vi "gun_const.vi"() -> (3 "Data Out":T1={"gun"={"num_lines"=0.0, "gain_kp1"=0.0, "gain_kp2"=0.0, "gain_ki"=0.0, "gain_kd"=0.0}, "turret"={"center_ana"=0.0, "volts_per_180"=0.0, "man_scale"=0.0, "turret_idg"={"low_fault_ana"=0.0, "high_fault_ana"=0.0, "min_ana"=0.0, "max_ana"=0.0, "movement_thresh"=0.0, "movement_time"=0.0}, "turret_pid"={"kP"=0.0, "kI"=0.0, "kD"=0.0}, "turret_invert"=TRUE, "turret_low_power"=0.0}, "tracking"={"velocity_lead_gain"=0.0, "velocity_rotation_gain"=0.0}, "hood"={"hood_idg"={"low_fault_ana"=0.0, "high_fault_ana"=0.0, "min_ana"=0.0, "max_ana"=0.0, "movement_thresh"=0.0, "movement_time"=0.0}, "hood_pid"={"kP"=0.0, "kI"=0.0, "kD"=0.0}, "hood_scale"={"min_ana"=0.0, "min_units"=0.0, "max_ana"=0.0, "max_units"=0.0}, "hood_invert"=FALSE}})   [LabVIEW 2011]
uses:
  gun_const_t.ctl
  gun_idg_const.ctl
  common/gain_const.ctl
  common/scale_const.ctl
  Robot Global Data.vi
panel:
  in  "data_practice":T1={"gun"={"num_lines"=4.0, "gain_kp1"=1.1e-05, "gain_kp2"=0.0015, "gain_ki"=0.00175, "gain_kd"=0.0055}, "turret"={"center_ana"=2.167, "volts_per_180"=-1.03, "man_scale"=0.0, "turret_idg"={"low_fault_ana"=0.4, "high_fault_ana"=3.3, "min_ana"=0.7, "max_ana"=3.07, "movement_thresh"=0.0, "movement_time"=1000.0}, "turret_pid"={"kP"=0.05, "kI"=0.0, "kD"=0.0}, "turret_invert"=TRUE, "turret_low_power"=0.2}, "tracking"={"velocity_lead_gain"=0.0, "velocity_rotation_gain"=0.0}, "hood"={"hood_idg"={"low_fault_ana"=3.0, "high_fault_ana"=5.6, "min_ana"=3.33, "max_ana"=5.0, "movement_thresh"=0.0, "movement_time"=0.0}, "hood_pid"={"kP"=0.3, "kI"=0.1, "kD"=0.0}, "hood_scale"={"min_ana"=3.33, "min_units"=67.0, "max_ana"=4.225, "max_units"=82.0}, "hood_invert"=TRUE}}
  in  "data_comp":T1={"gun"={"num_lines"=4.0, "gain_kp1"=1.1e-05, "gain_kp2"=0.0015, "gain_ki"=0.00175, "gain_kd"=0.0055}, "turret"={"center_ana"=2.15, "volts_per_180"=-1.03, "man_scale"=0.0, "turret_idg"={"low_fault_ana"=0.5, "high_fault_ana"=3.3, "min_ana"=0.8, "max_ana"=3.07, "movement_thresh"=0.0, "movement_time"=1000.0}, "turret_pid"={"kP"=0.05, "kI"=0.0, "kD"=0.0}, "turret_invert"=TRUE, "turret_low_power"=0.2}, "tracking"={"velocity_lead_gain"=0.0, "velocity_rotation_gain"=0.0}, "hood"={"hood_idg"={"low_fault_ana"=0.5, "high_fault_ana"=4.2, "min_ana"=1.6, "max_ana"=3.855, "movement_thresh"=0.0, "movement_time"=0.0}, "hood_pid"={"kP"=0.3, "kI"=0.1, "kD"=0.0}, "hood_scale"={"min_ana"=1.6, "min_units"=67.0, "max_ana"=2.74, "max_units"=81.0}, "hood_invert"=FALSE}}
  # "Orig Settings\nkp .002\nki 6e-5\n\nPID\nP .01\nI .00175\nD 0.1"
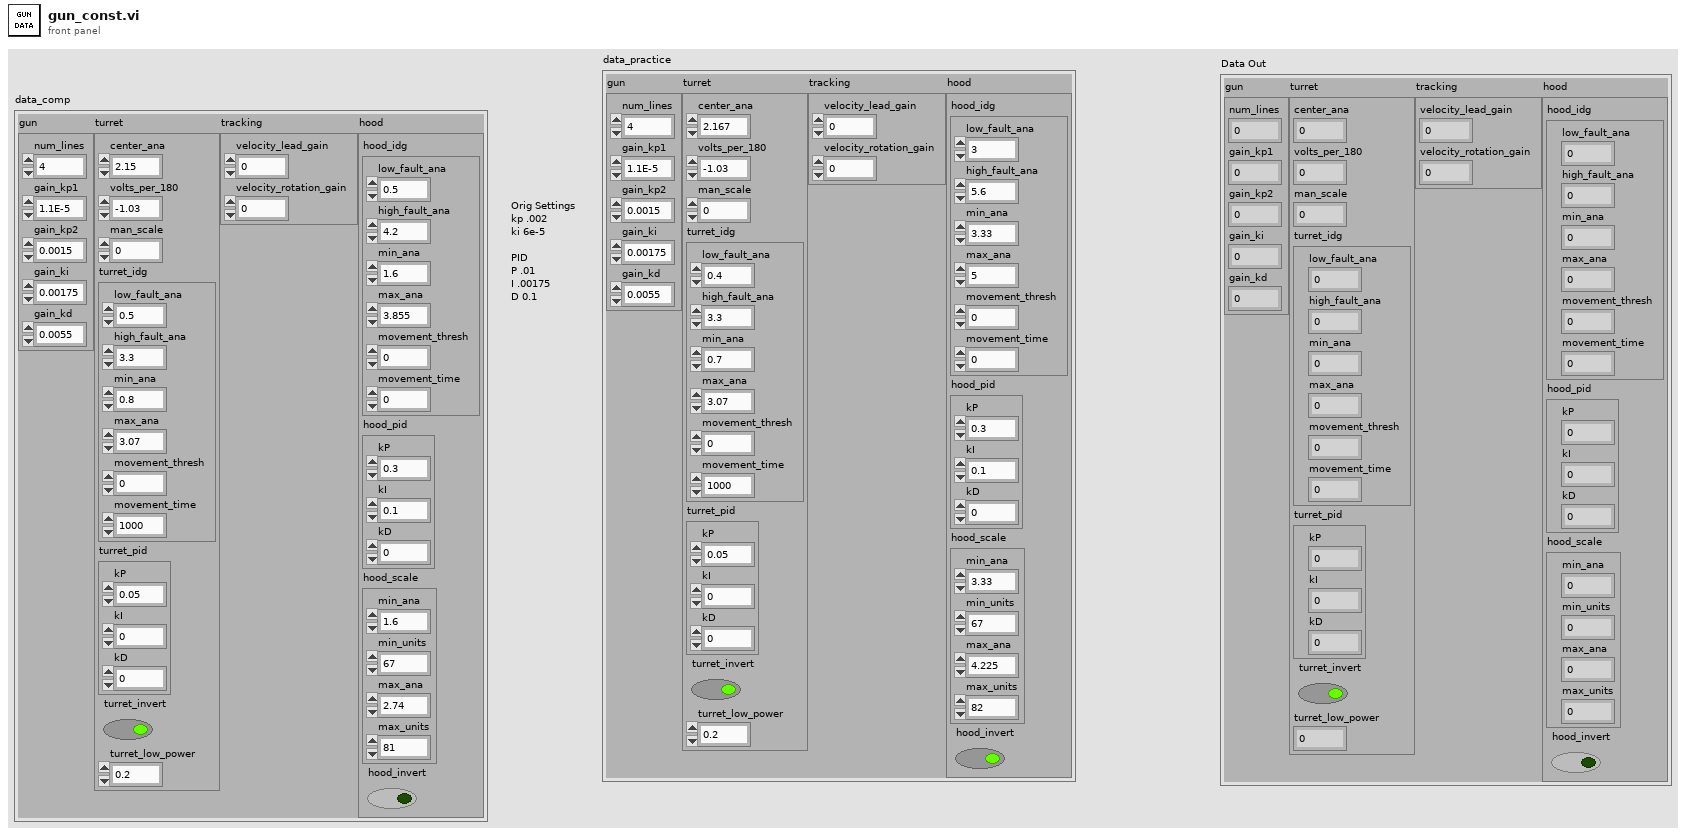
[diagram p1: front panel]
types:
  T1 = typedef "gun_const_t.ctl" = cluster{"gun":cluster{"num_lines":dbl, "gain_kp1":dbl, "gain_kp2":dbl, "gain_ki":dbl, "gain_kd":dbl}, "turret":cluster{"center_ana":dbl, "volts_per_180":dbl, "man_scale":dbl, "turret_idg":T2, "turret_pid":T3, "turret_invert":bool, "turret_low_power":dbl}, "tracking":cluster{"velocity_lead_gain":dbl, "velocity_rotation_gain":dbl}, "hood":cluster{"hood_idg":T2, "hood_pid":T3, "hood_scale":T4, "hood_invert":bool}}
  T2 = typedef "gun_idg_const.ctl" = cluster{"low_fault_ana":dbl, "high_fault_ana":dbl, "min_ana":dbl, "max_ana":dbl, "movement_thresh":dbl, "movement_time":dbl}
  T3 = typedef "gain_const.ctl" = cluster{"kP":dbl, "kI":dbl, "kD":dbl}
  T4 = typedef "scale_const.ctl" = cluster{"min_ana":dbl, "min_units":dbl, "max_ana":dbl, "max_units":dbl}
  T5 = typedef "Robot Ctl.ctl" = enum16{"Competition", "Practice"}
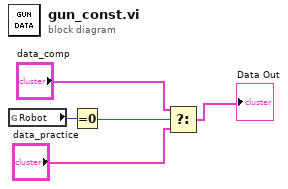
[diagram p0: block diagram]
diagram:
  n1 = global read "Robot Global Data.vi" "Robot"() -> (w5:T5)
  n2 = Equal To 0?(x=w5) -> (x = 0?=w4:bool)
  n3 = Select(t="data_comp", s=w4, f="data_practice") -> (s? t:f=→"Data Out":T1)
